vi "Read RT-BC Message.vi"(0 "transfer handle":u32, 11 "error in (no error)":errorcluster, 12 "Bus Section":T1) -> (4 "data buffer out":u16[](array[numeric]), 6 "status data out":u32[](array[numeric]), 8 "Data Available":bool, 15 "error out":errorcluster)   [LabVIEW 2013, in "AIT 1553 Custom Device.lvlib"]
uses:
  AIT 1553 Custom Device.lvlib
  RT Controls/AIT 1553 - Bus Section.ctl
  <instrlib>/AIT 1553/AIT 1553.lvlib
  <userlib>/MIL-STD-1553/Owl1553.lvlib
  <vilib>/NI Veristand/Custom Device Tools/Custom Device Utility Library/Custom Device Utility Library.lvlib
  <vilib>/NI Veristand/Custom Device Tools/Custom Device Utility Library/RT Debug String Color Spec.ctl
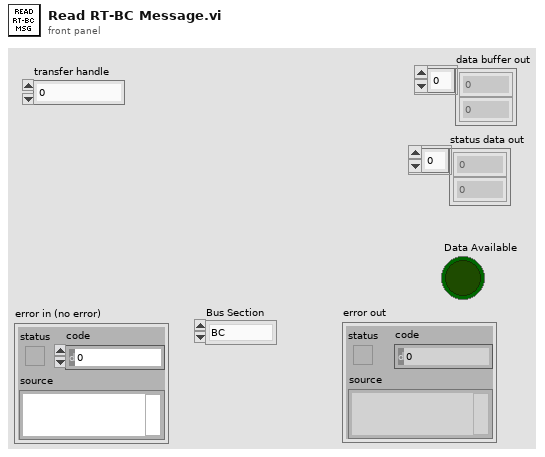
[diagram p1: front panel]
types:
  T1 = typedef "AIT 1553 Custom Device.lvlib/AIT 1553 - Bus Section.ctl" = enum16{"BC", "BM", "RT"}
  T2 = enum16{"OWL1553_BC_NO_TRANSFER_ERROR", "OWL1553_BC_CODING_OR_FRAMING_ERROR", "OWL1553_BC_STATUS_WORD_NOT_RECEIVED_ERROR", "OWL1553_BC_STATUS_WORD2_NOT_RECEIVED_ERROR", "OWL1553_BC_COULD_NOT_DETERMINE_ERROR"}
  T3 = enum16{"OWL1553_RT_NO_TRANSFER_ERROR", "OWL1553_RT_CODING_OR_FRAMING_ERROR", "OWL1553_RT_RESPONSE_TIMEOUT_ERROR", "OWL1553_RT_COULD_NOT_DETERMINE_ERROR"}
  T4 = typedef "Custom Device Utility Library.lvlib/RT Debug String Color Spec.ctl" = u16
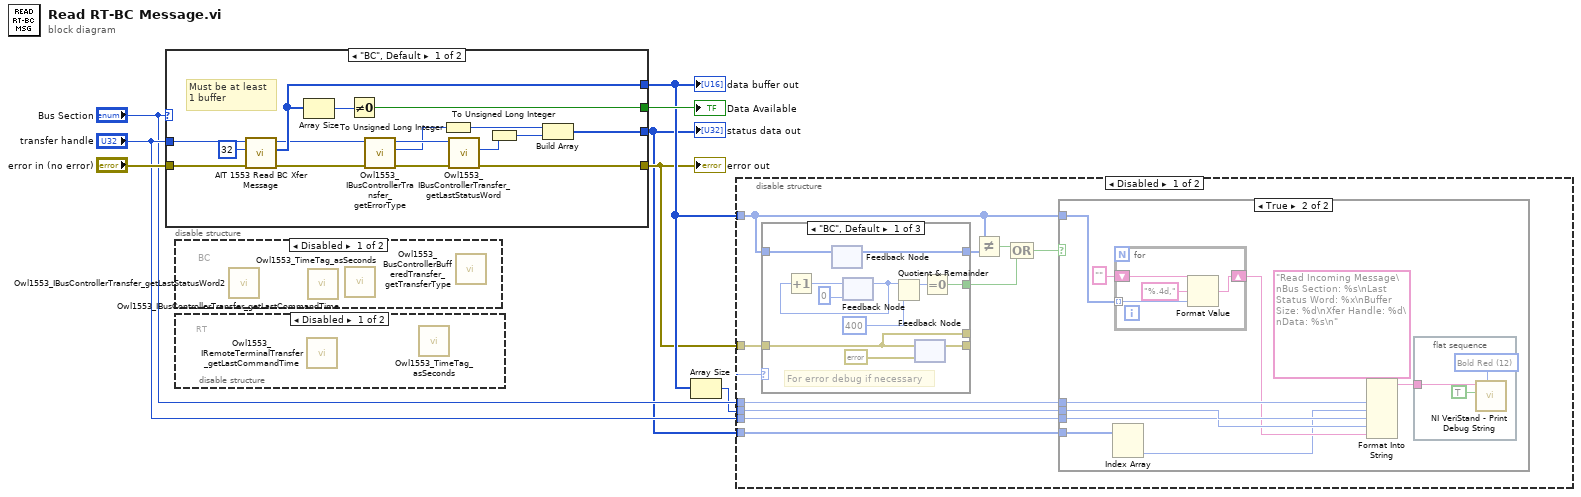
[diagram p0: block diagram]
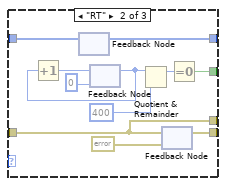
[diagram p4: hidden frame]
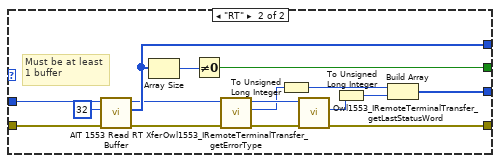
[diagram p8: hidden frame]
diagram:
  n1 = case shown="\"BC\", Default" "Bus Section" {
    tunnel: [w14 w30] -> w3
    tunnel: "error in (no error)" -> [w24 w37]
    tunnel: "transfer handle" -> [w22 w38]
    tunnel: [w23 w40] -> w7
    tunnel: [w21 w39] -> w5
    tunnel: [w11 w27] -> w1
    frame "BC", Default {
      # "Must be at least \n1 buffer"
      n2 = call <instrlib>:"AIT 1553 Read BC Xfer Message.vi"("error in"=w24, "buffer size"=u32 32, "BC transfer handle in"=w22) -> ("error out"=w18:errorcluster, "data buffer out"=w21:u16[], "BC transfer handle out"=w17:u32)  [unwired: 6 in]
      n3 = Array Size(array=w21) -> (size(s)=w19:i32)
      n4 = Not Equal To 0?(x=w19) -> (x != 0?=w23:bool)
      n5 = call <userlib>:"Owl1553_IBusControllerTransfer_getErrorType.vi"("error in (no error)"=w18, "transfer handle"=w17) -> ("error out"=w16:errorcluster, "error report type"=w13:T2, "transfer handle"=w15:u32)  [unwired: 7 in]
      n6 = To Unsigned Long Integer(number=w13) -> (unsigned 32bit integer=w10:u32)
      n7 = call <userlib>:"Owl1553_IBusControllerTransfer_getLastStatusWord.vi"("error in (no error)"=w16, "transfer handle"=w15) -> ("error out"=w14:errorcluster, "last status word"=w12:u16)  [unwired: 7 in, 1 out]
      n8 = To Unsigned Long Integer(number=w12) -> (unsigned 32bit integer=w9:u32)
      n9 = Build Array(w10, w9) -> (w11:u32[])
    }
    frame "RT" {
      # "Must be at least\n1 buffer"
      n10 = call <instrlib>:"AIT 1553 Read RT Xfer Buffer.vi"("error in"=w37, "word count in"=u32 32, "RT transfer handle in"=w38) -> ("error out"=w33:errorcluster, "buffer out"=w39:u16[], "RT transfer handle out"=w34:u32)  [unwired: 6 in]
      n11 = Array Size(array=w39) -> (size(s)=w35:i32)
      n12 = Not Equal To 0?(x=w35) -> (x != 0?=w40:bool)
      n13 = call <userlib>:"Owl1553_IRemoteTerminalTransfer_getErrorType.vi"("error in (no error)"=w33, "transfer handle"=w34) -> ("error out"=w31:errorcluster, "error type"=w29:T3, "transfer handle"=w32:u32)  [unwired: 7 in]
      n14 = To Unsigned Long Integer(number=w29) -> (unsigned 32bit integer=w26:u32)
      n15 = call <userlib>:"Owl1553_IRemoteTerminalTransfer_getLastStatusWord.vi"("error in (no error)"=w31, "transfer handle"=w32) -> ("error out"=w30:errorcluster, "status word"=w28:u16)  [unwired: 7 in, 1 out]
      n16 = To Unsigned Long Integer(number=w28) -> (unsigned 32bit integer=w25:u32)
      n17 = Build Array(w26, w25) -> (w27:u32[])
    }
  }
  "error out" <- w3
  "Data Available" <- w7
  "data buffer out" <- w5
  "status data out" <- w1
  n18 = disable-structure shown="Disabled" {
    frame Disabled {
      # "BC"
      n19 = call <userlib>:"Owl1553_IBusControllerTransfer_getLastStatusWord2.vi"() -> ()  [unwired: 9 in, 3 out]
      n20 = call <userlib>:"Owl1553_IBusControllerTransfer_getLastCommandTime.vi"() -> ()  [unwired: 9 in, 3 out]
      n21 = call <userlib>:"Owl1553_TimeTag_asSeconds.vi"() -> ()  [unwired: 9 in, 3 out]
      n22 = call <userlib>:"Owl1553_BusControllerBufferedTransfer_getTransferType.vi"() -> ()  [unwired: 7 in, 3 out]
    }
    frame Enabled {
    }
  }
  n23 = disable-structure shown="Disabled" {
    frame Disabled {
      # "RT"
      n24 = call <userlib>:"Owl1553_IRemoteTerminalTransfer_getLastCommandTime.vi"() -> ()  [unwired: 9 in, 3 out]
      n25 = call <userlib>:"Owl1553_TimeTag_asSeconds.vi"() -> ()  [unwired: 9 in, 3 out]
    }
    frame Enabled {
    }
  }
  n26 = Array Size(array=w5) -> (size(s)=w2:i32)
  n27 = disable-structure shown="Disabled" {
    disable-tunnel: "transfer handle" -> [w50 _]
    disable-tunnel: w5 -> [w47 _]
    disable-tunnel: "Bus Section" -> [w46 _]
    disable-tunnel: w3 -> [w45 _]
    disable-tunnel: w2 -> [w44 _]
    disable-tunnel: w1 -> [w41 _]
    frame Disabled {
      n28 = case shown="\"BC\", Default" w46 {
        tunnel: [w56 w67 _] -> w43
        tunnel: w47 -> [w55 w66 w73]
        tunnel: [w54 w65 w73] -> w48
        tunnel: [w51 w62 _] -> _
        tunnel: [w52 w63 _] -> _
        tunnel: w45 -> [w51 w62 _]
        frame "BC", Default {
          # "For error debug if necessary"
          n29 = feedback #1() -> (w54:u16[])  [unwired: 1 in]
          n30 = feedback-in #1(w55) -> ()
          n31 = feedback #2(0) -> (w57:i32)
          n32 = Increment(x=w57) -> (x+1=w59:i32)
          n33 = feedback-in #2(w59) -> ()
          n34 = Quotient & Remainder(x=w57, y=400) -> (x-y*floor(x/y)=w61:i32)  [unwired: 1 out]
          n35 = feedback #3(errorcluster {"status"=FALSE, "code"=0, "source"=""} ("error out")) -> (w52:errorcluster)
          n36 = feedback-in #3(w51) -> ()
          n37 = Equal To 0?(x=w61) -> (x = 0?=w56:bool)
        }
        frame "RT" {
          n38 = feedback #4() -> (w65:u16[])  [unwired: 1 in]
          n39 = feedback-in #4(w66) -> ()
          n40 = feedback #5(0) -> (w68:i32)
          n41 = Increment(x=w68) -> (x+1=w70:i32)
          n42 = feedback-in #5(w70) -> ()
          n43 = Quotient & Remainder(x=w68, y=400) -> (x-y*floor(x/y)=w72:i32)  [unwired: 1 out]
          n44 = feedback #6(errorcluster {"status"=FALSE, "code"=0, "source"=""} ("error out")) -> (w63:errorcluster)
          n45 = feedback-in #6(w62) -> ()
          n46 = Equal To 0?(x=w72) -> (x = 0?=w67:bool)
        }
        frame "BM" {
        }
      }
      n47 = Not Equal?(x=w47, y=w48) -> (x != y?=w49:bool)
      n48 = Compound Arithmetic op=OR(w49, w43) -> (w42:bool)
      n49 = case shown="True" w42 {
        tunnel: w46 -> [_ w81]
        tunnel: w44 -> [_ w80]
        tunnel: w47 -> [_ w79]
        tunnel: w50 -> [_ w77]
        tunnel: w41 -> [_ w75]
        frame False {
        }
        frame True {
          n50 = Index Array(array=w75) -> (element #2=w74:u32)  [unwired: 2 in, 1 out]
          n51 = for {
            tunnel: w79 -> [w84] mode=indexing
            shift-right: [w85] -> w76
            shift-left: "" ("format string") -> [w86]
            n52 = Format Value(string ("")=w86, format string="%.4d,", value (0)=w84) -> (output string=w85:string)
          }
          n53 = Format Into String(format string="Read Incoming Message\nBus Section: %s\nLast Status Word: %x\nBuffer Size: %d\nXfer Handle: %d\nData: %s\n", w81, w74, w80, w77, w76) -> (resulting string=w82:string)  [unwired: 2 in, 1 out]
          n54 = flat-sequence {
            tunnel: w82 -> [w88]
            frame #0 {
              w89 = T4 12 items=["Plain White"=7, "Bold White"=15, "Bold Blue"=9, "Bold Green"=10, "Bold Red"=12] ("Attribute")
              n55 = call <vilib>:"NI VeriStand - Print Debug String.vi"("Attribute"=w89, "Add to log file? (T)"=TRUE, "Message"=w88) -> ()  [unwired: 8 in, 1 out]
            }
          }
        }
      }
    }
    frame Enabled {
    }
  }
